vi "1.vi"() -> ()   [LabVIEW 2015]
panel:
  out "appended array":dbl[][](array[numeric])
  in  "Array":dbl[](array[numeric])
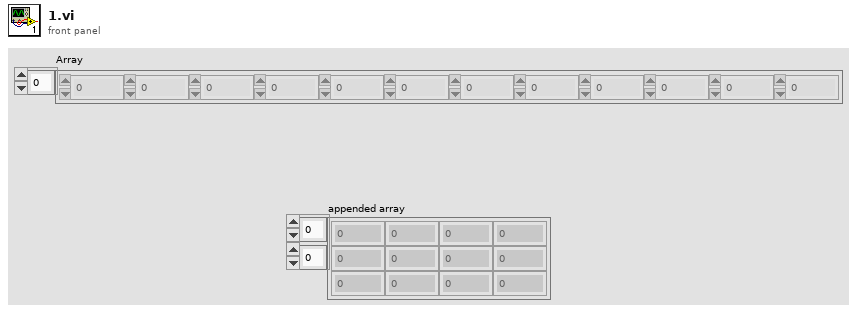
[diagram p1: front panel]
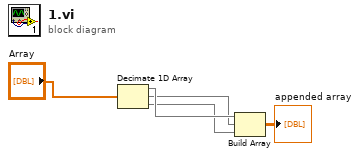
[diagram p0: block diagram]
diagram:
  n1 = Decimate 1D Array("Array") -> (w4:dbl[], w3:dbl[], w2:dbl[])
  n2 = Build Array(w4, w3, w2) -> (→"appended array":dbl[][])
